vi "Set Connector Pane State.vi"(8 "error in (no error)":errorcluster, 10 "callers adapt? (true)":bool=TRUE, 11 "PPL in":refnum<class "NI_AB_API_PPL.lvclass">) -> (0 "error out":errorcluster, 3 "PPL out":refnum<class "NI_AB_API_PPL.lvclass">)   [LabVIEW 2020, in "NI_AB_API_PPL.lvclass"]
uses:
  <vilib>/AppBuilder/AB_API/PPL/NI_AB_API_PPL.lvclass
  e:/builds/penguin/labview/branches/2020/dev/dist/vi.lib/AppBuilder/AB_API/Build/NI_AB_API_Build.lvclass
  <vilib>/AppBuilder/AB_Classes/PackedLib/AB_PackedLibrary.lvclass
  e:/builds/penguin/labview/branches/2020/dev/dist/vi.lib/AppBuilder/AB_Classes/Build/AB_Build.lvclass
  <vilib>/AppBuilder/AB_API/PPL/NI_AB_API_PPL.lvclass/NI_AB_API_PPL.ctl
  <vilib>/AppBuilder/AB_API/Build/NI_AB_API_Build.lvclass
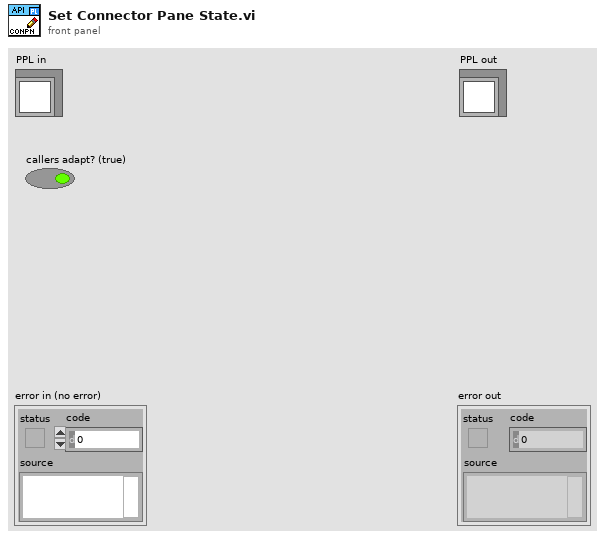
[diagram p1: front panel]
types:
  T1 = typedef "AB_PackedLibrary.ctl" = cluster{"callersAdapt":bool, "showWarnings":bool, "verifyConnpane":bool, "eng_sourceLibrary":string, "eng_packedLib_inMemory":bool}
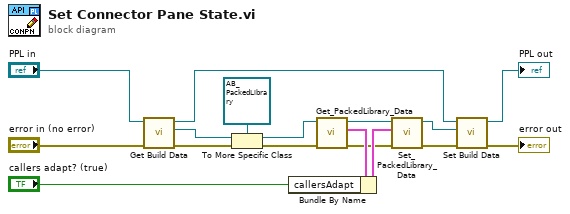
[diagram p0: block diagram]
diagram:
  n1 = call <vilib>:"Get Build Data.vi"("error in (no error)"="error in (no error)", "NI_AB_API_Build in"="PPL in") -> ("error out"=w4:errorcluster, "AB_Build.lvclass"=w5:refnum<class "AB_Build.lvclass">, "NI_AB_API_Build out"=w9:refnum<class "NI_AB_API_PPL.lvclass">)  [unwired: 7 in]
  n2 = To More Specific Class(target class=refnum<class "AB_PackedLibrary.lvclass"> refnum ("AB_PackedLibrary.lvclass"), reference=w5, error in=w4) -> (specific class reference=w6:refnum<class "AB_PackedLibrary.lvclass">, error out=w3:errorcluster)
  n3 = call <vilib>:"Get_PackedLibrary_Data.vi"("error in (no error)"=w3, "Class in"=w6) -> ("error out"=w2:errorcluster, "data"=w11:T1, "Class out"=w12:refnum<class "AB_PackedLibrary.lvclass">)  [unwired: 7 in]
  n4 = Bundle By Name(cluster=w11, "callersAdapt"="callers adapt? (true)") -> (w10:T1)
  n5 = call <vilib>:"Set_PackedLibrary_Data.vi"("error in (no error)"=w2, "data"=w10, "Class in"=w12) -> ("error out"=w1:errorcluster, "Class out"=w8:refnum<class "AB_PackedLibrary.lvclass">)  [unwired: 7 in]
  n6 = call <vilib>:"Set Build Data.vi"("error in (no error)"=w1, "AB_Build.lvclass"=w8, "NI_AB_API_Build in"=w9) -> ("error out"=→"error out":errorcluster, "NI_AB_API_Build out"=→"PPL out":refnum<class "NI_AB_API_PPL.lvclass">)  [unwired: 7 in]
